vi "Auto Drive Back.vi"(10 "Distance":dbl, 11 "Execute?":bool) -> (3 "Done":bool)   [LabVIEW 2012]
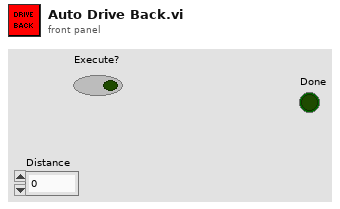
[diagram p1: front panel]
types:
  T1 = typedef "WPI_EncoderDevRef.ctl" = cluster{"DevStatus":errorcluster, "EncoderIndex":T2, "CounterIndex":T3, "DistancePerCount":dbl, "Decoding Type":T4}
  T2 = typedef "FPGA_EncoderIdx.ctl" = enum8{"Enc 0", "Enc 1", "Enc 2", "Enc 3", "Invalid"}
  T3 = typedef "FPGA_CounterCtrSystemIndex.ctl" = enum8{"Ctr 0", "Ctr 1", "Ctr 2", "Ctr 3", "Ctr 4", "Ctr 5", "Ctr 6", "Ctr 7", "Invalid"}
  T4 = typedef "WPI_EncoderType.ctl" = enum16{"1x", "2x", "4x"}
  T5 = typedef "WPI_MotorControlDeviceRef.ctl" = cluster{"DeviceStatus":errorcluster, "Type":enum16{"PWM", "CAN"}, "PWM":cluster{"Digital Module":T6, "PWM Channel":T7, "DeadBand":T8}, "CAN":cluster{"Device Number":u8, "Control Mode":T9, "Semaphore":T10, "Max Vout":dbl}, "Invert":bool, "TransformRef":T11, "InvTransformRef":T11}
  T6 = typedef "FPGA_TypedefDigitalModule.ctl" = enum16{"Digital Module 1", "Digital Module 2"}
  T7 = typedef "FPGA_DIOPWMChannel.ctl" = enum8{"PWM 1", "PWM 2", "PWM 3", "PWM 4", "PWM 5", "PWM 6", "PWM 7", "PWM 8", "PWM 9", "PWM 10", "Invalid"}
  T8 = typedef "WPI_PWMDeadband.ctl" = cluster{"Name":string, "maxPositivePwm":i32, "minPositivePwm":i32, "centerPwm":i32, "maxNegativePwm":i32, "minNegativePwm":i32, "angularRange":u16}
  T9 = typedef "WPI_CANJaguar_ControlMode.ctl" = enum8{"Percent VBus", "Current", "Speed", "Position", "Voltage"}
  T10 = typedef "Semaphore RefNum" = refnum<k1>
  T11 = typedef "WPI_PWMTransform_ConPane.ctl" = refnum<vi>
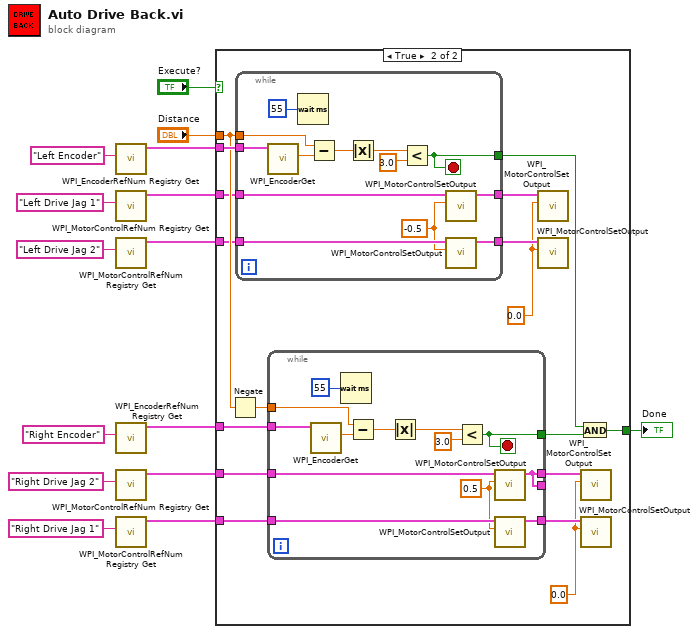
[diagram p0: block diagram]
diagram:
  n1 = call <vilib>:"WPI_EncoderRefNum Registry Get.vi"("refnum name"="Left Encoder") -> ("EncoderDevRef"=w3:T1)  [unwired: 9 in, 1 out]
  n2 = call <vilib>:"WPI_MotorControlRefNum Registry Get.vi"("refnum name"="Left Drive Jag 1") -> ("MotorControlDevRef"=w4:T5)  [unwired: 9 in, 1 out]
  n3 = call <vilib>:"WPI_MotorControlRefNum Registry Get.vi"("refnum name"="Left Drive Jag 2") -> ("MotorControlDevRef"=w5:T5)  [unwired: 9 in, 1 out]
  n4 = call <vilib>:"WPI_EncoderRefNum Registry Get.vi"("refnum name"="Right Encoder") -> ("EncoderDevRef"=w1:T1)  [unwired: 9 in, 1 out]
  n5 = call <vilib>:"WPI_MotorControlRefNum Registry Get.vi"("refnum name"="Right Drive Jag 2") -> ("MotorControlDevRef"=w7:T5)  [unwired: 9 in, 1 out]
  n6 = call <vilib>:"WPI_MotorControlRefNum Registry Get.vi"("refnum name"="Right Drive Jag 1") -> ("MotorControlDevRef"=w6:T5)  [unwired: 9 in, 1 out]
  n7 = case shown="True" "Execute?" {
    selector: "Execute?" -> [w16 _]
    tunnel: [w16 w23] -> w8
    tunnel: w7 -> [_ w28]
    tunnel: w6 -> [_ w27]
    tunnel: w5 -> [_ w29]
    tunnel: w4 -> [_ w26]
    tunnel: w3 -> [_ w33]
    tunnel: "Distance" -> [_ w32]
    tunnel: w1 -> [_ w30]
    frame False {
    }
    frame True {
      w17 = 0.0 ("Output")
      w18 = 0.0 ("Output")
      n8 = Negate(x=w32) -> (-x=w31:dbl)
      n9 = while {
        tunnel: w33 -> [w59]
        tunnel: w32 -> [w57]
        tunnel: w26 -> [w52]
        tunnel: w29 -> [w51]
        tunnel: [w49] -> w25
        tunnel: [w48] -> w20
        tunnel: [w47] -> w19
        stop <- w49 stop-if-true
        w50 = -0.5 ("Output")
        n10 = call <vilib>:"WPI_EncoderGet.vi"("EncoderDevRef"=w59) -> ("Distance"=w56:dbl)  [unwired: 5 in, 5 out]
        n11 = Wait (ms)(milliseconds to wait=u32 55) -> ()  [unwired: 1 out]
        n12 = Subtract(x=w57, y=w56) -> (x-y=w58:dbl)
        n13 = Absolute Value(x=w58) -> (abs(x)=w55:dbl)
        n14 = Less?(x=w55, y=3.0) -> (x < y?=w49:bool)
        n15 = call <vilib>:"WPI_MotorControlSetOutput.vi"("Output"=w50, "MotorControlDevRef"=w52) -> ("MotorControlDevRef"=w47:T5)  [unwired: 7 in, 2 out]
        n16 = call <vilib>:"WPI_MotorControlSetOutput.vi"("Output"=w50, "MotorControlDevRef"=w51) -> ("MotorControlDevRef"=w48:T5)  [unwired: 7 in, 2 out]
      }
      n17 = while {
        tunnel: w30 -> [w46]
        tunnel: w31 -> [w44]
        tunnel: w28 -> [w39]
        tunnel: w27 -> [w38]
        tunnel: [w36] -> w24
        tunnel: [w35] -> w22
        tunnel: [w35] -> _
        tunnel: [w34] -> w21
        stop <- w36 stop-if-true
        w37 = 0.5 ("Output")
        n18 = call <vilib>:"WPI_EncoderGet.vi"("EncoderDevRef"=w46) -> ("Distance"=w43:dbl)  [unwired: 5 in, 5 out]
        n19 = Wait (ms)(milliseconds to wait=u32 55) -> ()  [unwired: 1 out]
        n20 = Subtract(x=w44, y=w43) -> (x-y=w45:dbl)
        n21 = Absolute Value(x=w45) -> (abs(x)=w42:dbl)
        n22 = Less?(x=w42, y=3.0) -> (x < y?=w36:bool)
        n23 = call <vilib>:"WPI_MotorControlSetOutput.vi"("Output"=w37, "MotorControlDevRef"=w39) -> ("MotorControlDevRef"=w35:T5)  [unwired: 7 in, 2 out]
        n24 = call <vilib>:"WPI_MotorControlSetOutput.vi"("Output"=w37, "MotorControlDevRef"=w38) -> ("MotorControlDevRef"=w34:T5)  [unwired: 7 in, 2 out]
      }
      n25 = call <vilib>:"WPI_MotorControlSetOutput.vi"("Output"=w18, "MotorControlDevRef"=w19) -> ()  [unwired: 7 in, 3 out]
      n26 = call <vilib>:"WPI_MotorControlSetOutput.vi"("Output"=w18, "MotorControlDevRef"=w20) -> ()  [unwired: 7 in, 3 out]
      n27 = And(x=w25, y=w24) -> (x .and. y?=w23:bool)
      n28 = call <vilib>:"WPI_MotorControlSetOutput.vi"("Output"=w17, "MotorControlDevRef"=w22) -> ()  [unwired: 7 in, 3 out]
      n29 = call <vilib>:"WPI_MotorControlSetOutput.vi"("Output"=w17, "MotorControlDevRef"=w21) -> ()  [unwired: 7 in, 3 out]
    }
  }
  "Done" <- w8
